vi "读tdms.vi"(8 "错误输入（无错误）":errorcluster, 11 "引用句柄输入":refnum<k34>) -> (0 "错误输出":errorcluster, 1 "数据":sgl[](array[numeric]), 2 "添加的数组":sgl[][](array[numeric]), 3 "引用句柄输出":refnum<k34>)   [LabVIEW 2012]
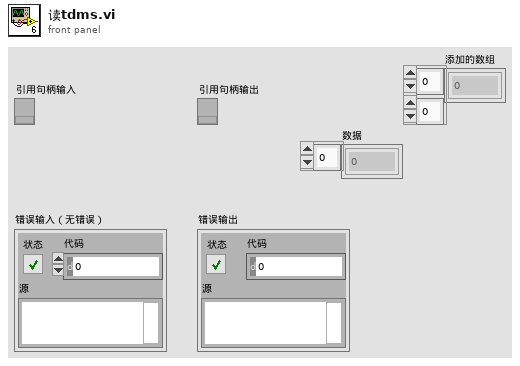
[diagram p1: front panel]
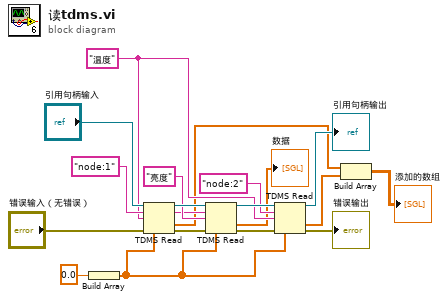
[diagram p0: block diagram]
diagram:
  w8 = "温度"
  n1 = Build Array(sgl 0.0) -> (w7:sgl[])
  n2 = TDMS Read(0:"引用句柄输入", 5:"node:1" ("组名称输入"), 7:w8, 11:"错误输入（无错误）", 12:w7) -> (4:w15:refnum<k34>, 6:w9:string, 10:w3:sgl[], 15:w14:errorcluster)  [unwired: 3 in, 2 out]
  n3 = TDMS Read(0:w15, 5:w9, 7:"亮度", 11:w14, 12:w7) -> (4:w12:refnum<k34>, 10:→"数据":sgl[], 15:w11:errorcluster)  [unwired: 3 in, 3 out]
  n4 = TDMS Read(0:w12, 5:"node:2" ("组名称输入"), 7:w8, 11:w11, 12:w7) -> (4:→"引用句柄输出":refnum<k34>, 10:w2:sgl[], 15:→"错误输出":errorcluster)  [unwired: 3 in, 3 out]
  n5 = Build Array(w3, w2) -> (→"添加的数组":sgl[][])
